vi "Format Aquisition Sequence Array.vi"(8 "Capture/Live":string, 11 "Sequence Cluster Array":T1[](array[typedef]) {"Image Acquisition Parameters"."Z Steps Size (um)" min=0.0; "Image Acquisition Parameters"."Number of Z Steps" min=1; "Image Acquisition Parameters"."Frames Accumulations" min=1; "Image Acquisition Parameters"."Frames Per Capture" min=1; "Image Acquisition Parameters"."Line Accumulations" min=1; "Image Acquisition Parameters"."Image Format" items=["64 x 64"=64, "128 x 128"=128, "256 x 256"=256, "512 x 512"=512, "1024 x 1024"=1024, "2048 x 2048"=2048]; "Laser Parameters"."405 Power (0-5V)" min=0.0 max=5.0}) -> (0 "Channel pixel size array":cluster{i32, i32}[](array[cluster]), 1 "Number of Channels":i32, 2 "Image Acquisition Parameter Array":T2[](array[typedef]) {"Z Steps Size (um)" min=0.0; "Number of Z Steps" min=1; "Frames Accumulations" min=1; "Frames Per Capture" min=1; "Line Accumulations" min=1; "Image Format" items=["64 x 64"=64, "128 x 128"=128, "256 x 256"=256, "512 x 512"=512, "1024 x 1024"=1024, "2048 x 2048"=2048]}, 3 "Detector Parameters Array":T4[](array[typedef]), 4 "Channel Acquisition Parameters Array":T2[](array[typedef]) {"Z Steps Size (um)" min=0.0; "Number of Z Steps" min=1; "Frames Accumulations" min=1; "Frames Per Capture" min=1; "Line Accumulations" min=1; "Image Format" items=["64 x 64"=64, "128 x 128"=128, "256 x 256"=256, "512 x 512"=512, "1024 x 1024"=1024, "2048 x 2048"=2048]})   [LabVIEW 2016]
uses:
  Detectors.ctl
  Type Defs/Image Acquisition Parameters.ctl
  Sequence Cluster_Ctrl.ctl
  Laser Controls.ctl
panel:
  # "Copyright (C) 2020 Edward S Allgeyer\n\nRedistribution and use in source and binary forms, with or without\nmodification, are permitted provided that the following conditions\nare met:\n\n1. Redistributions of source code must retain the above copyright\n   notice, this list of conditions and the following disclaimer.\n\n2. Redistributions in binary form must reproduce the above copyright\n   notice, this list of conditions and the following disclaimer in\n   the documentation and/or other materials provided with the\n   distribution.\n\n3. Neither the name of the copyright holder nor the names of its\n   contributors may be used to endorse or promote products derived\n   from this software without specific prior written permission.\n\nTHIS SOFTWARE IS PROVIDED BY THE COPYRIGHT HOLDERS AND CONTRIBUTORS\n\"AS IS\" AND ANY EXPRESS OR IMPLIED WARRANTIES, INCLUDING, BUT NOT\nLIMITED TO, THE IMPLIED WARRANTIES OF MERCHANTABILITY AND FITNESS\nFOR A PARTICULAR PURPOSE ARE DISCLAIMED. IN NO EVENT SHALL THE\nCOPYRIGHT HOLDER OR CONTRIBUTORS BE LIABLE FOR ANY DIRECT, INDIRECT,\nINCIDENTAL, SPECIAL, EXEMPLARY, OR CONSEQUENTIAL DAMAGES (INCLUDING,\nBUT NOT LIMITED TO, PROCUREMENT OF SUBSTITUTE GOODS OR SERVICES;\nLOSS OF USE, DATA, OR PROFITS; OR BUSINESS INTERRUPTION) HOWEVER\nCAUSED AND ON ANY THEORY OF LIABILITY, WHETHER IN CONTRACT, STRICT\nLIABILITY, OR TORT (INCLUDING NEGLIGENCE OR OTHERWISE) ARISING IN\nANY WAY OUT OF THE USE OF THIS SOFTWARE, EVEN IF ADVISED OF THE\nPOSSIBILITY OF SUCH DAMAGE."
  # "XY"
  # "Z"
  # "Length"
  # "Height"
  # "XY"
  # "Z"
  # "Length"
  # "Height"
  # "XY"
  # "Z"
  # "Length"
  # "Height"
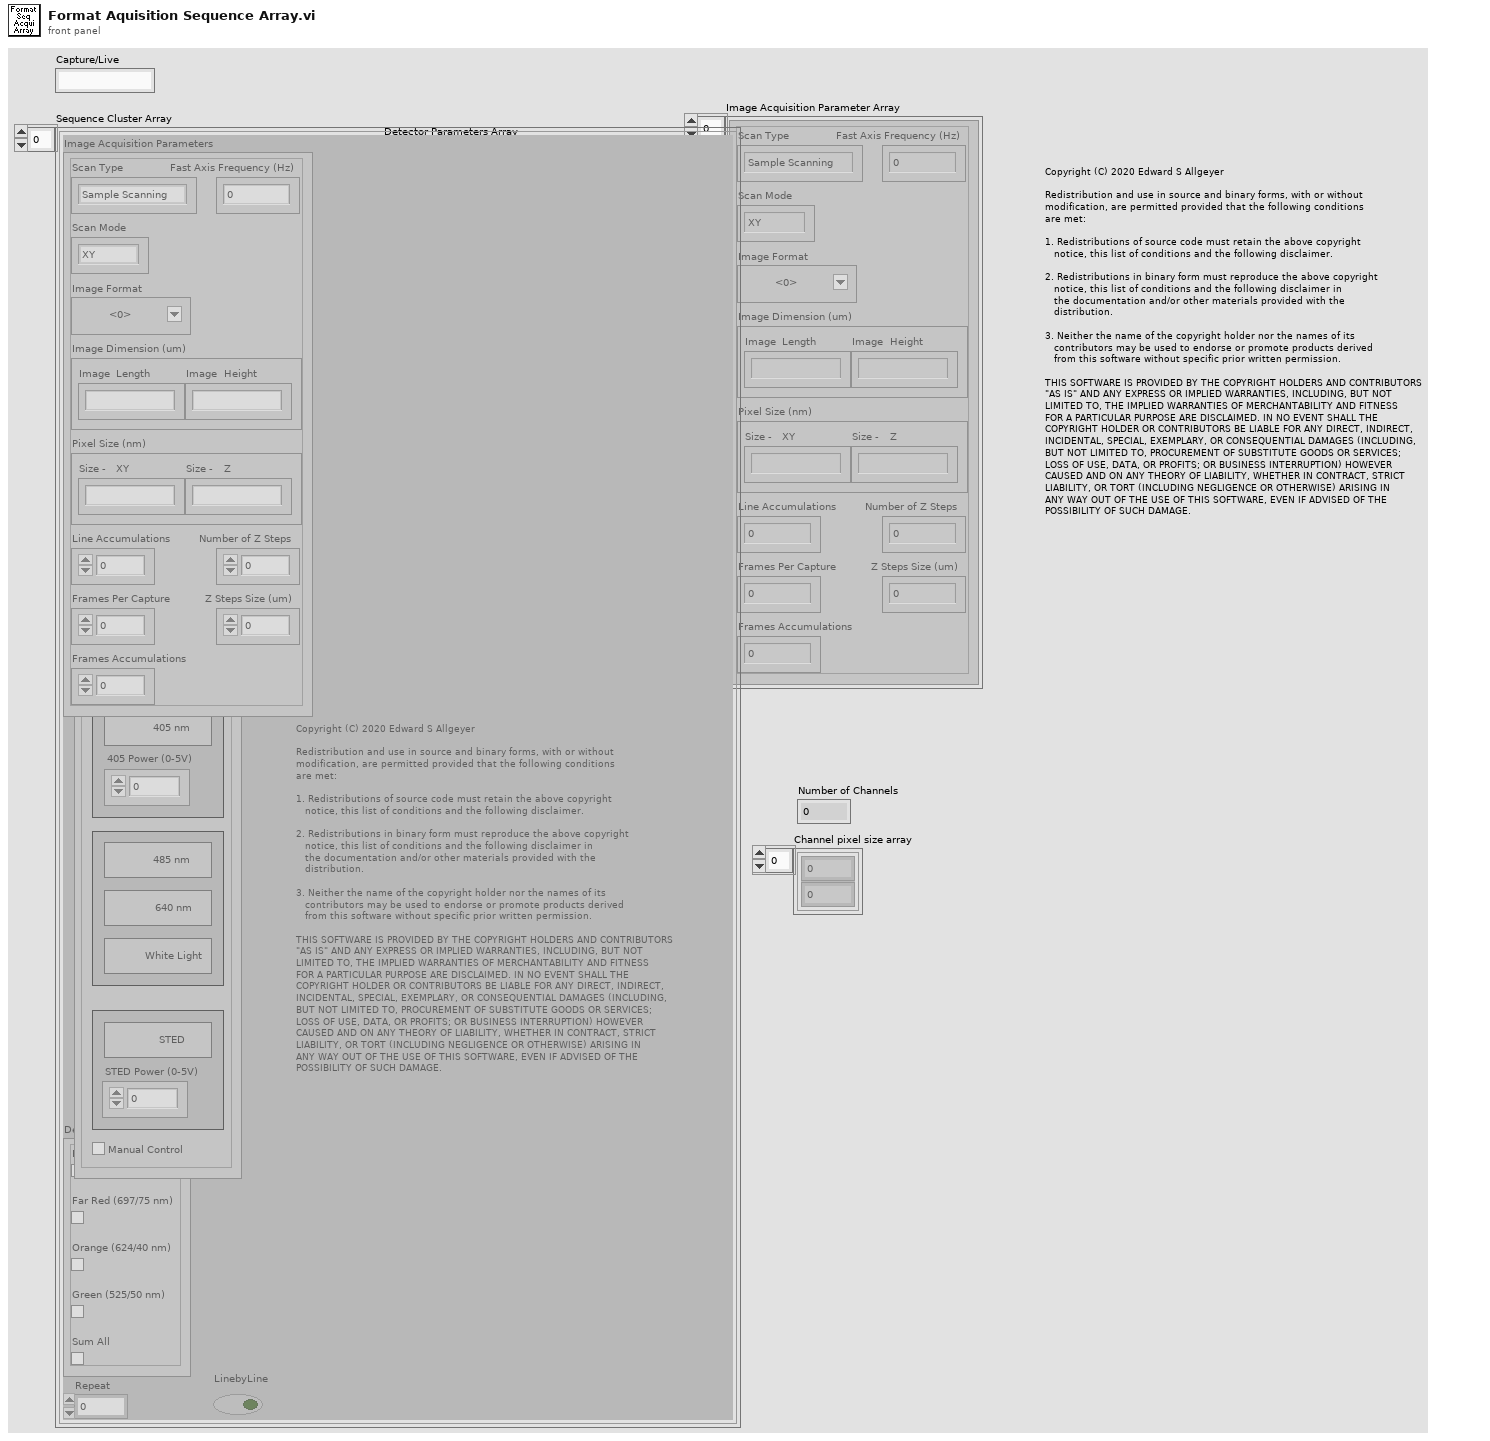
[diagram p1: front panel]
types:
  T1 = typedef "Sequence Cluster_Ctrl.ctl" = cluster{"Image Acquisition Parameters":T2, "Laser Parameters":T3, "Detectors Parameters":T4, "Repeat":dbl, "LinebyLine":bool}
  T2 = typedef "Image Acquisition Parameters.ctl" = cluster{"Scan Type":enum16{"Sample Scanning", "Beam Scanning"}, "Scan Mode":enum16{"XY", "XZ", "YZ", "XYZ"}, "Fast Axis Frequency (Hz)":dbl, "Image Format":u16, "Line Accumulations":u16, "Frames Per Capture":u16, "Frames Accumulations":u16, "Image Dimension (um)":dbl[], "Number of Z Steps":u8, "Z Steps Size (um)":dbl, "Pixel Size (nm)":dbl[]}
  T3 = typedef "Laser Controls.ctl" = cluster{"STED Power (0-5V)":dbl, "STED":bool, "640 nm":bool, "485 nm":bool, "Manual Control":bool, "White Light":bool, "405 nm":bool, "405 Power (0-5V)":dbl}
  T4 = typedef "Detectors.ctl" = cluster{"PMT":bool, "Far Red (697/75 nm)":bool, "Orange (624/40 nm)":bool, "Green (525/50 nm)":bool, "Sum All":bool}
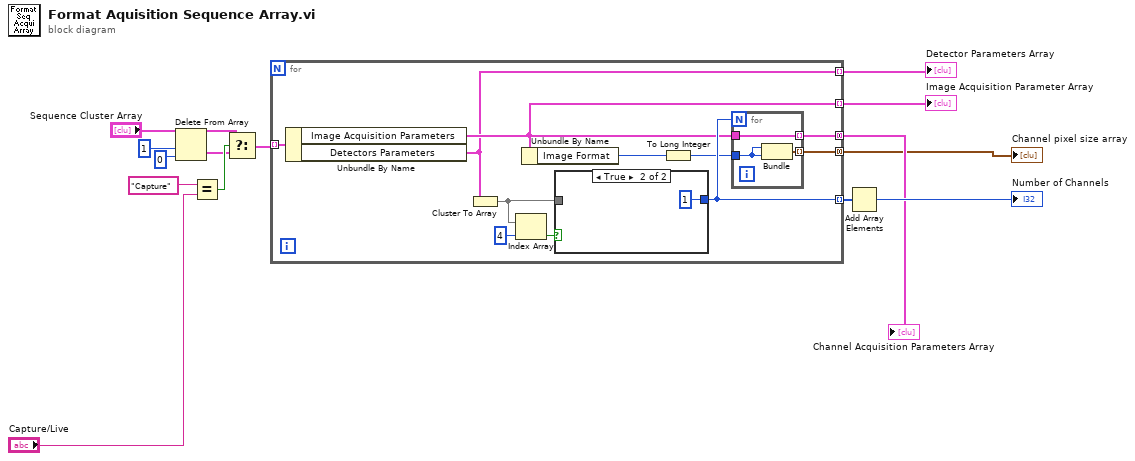
[diagram p0: block diagram]
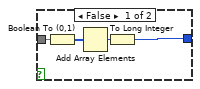
[diagram p2: hidden frame]
diagram:
  n1 = Delete From Array(array="Sequence Cluster Array", length=1, index=0) -> (deleted portion=w9:T1[], array with subset deleted=w8:T1[])
  n2 = Equal?(x="Capture" ("Action"), y="Capture/Live") -> (x = y?=w11:bool)
  n3 = Select(t=w8, s=w11, f=w9) -> (s? t:f=w10:T1[])
  n4 = for {
    tunnel: w10 -> [w26] mode=indexing
    tunnel: [w22] -> w5 mode=concatenating
    tunnel: [w23] -> w4 mode=indexing
    tunnel: [w21] -> w14 mode=indexing
    tunnel: [w20] -> w12 mode=concatenating
    tunnel: [w16] -> w15 mode=indexing
    n5 = Unbundle By Name(w26) -> ("Image Acquisition Parameters"=w21:T2, "Detectors Parameters"=w16:T4)
    n6 = Cluster To Array(cluster=w16) -> (array=w24:bool[])
    n7 = Index Array(array=w24, index=4) -> (element=w17:bool)
    n8 = Unbundle By Name(w21) -> ("Image Format"=w19:u16)
    n9 = case shown="True" w17 {
      tunnel: w24 -> [w30 _]
      tunnel: [w29 1] -> w23
      frame False {
        n10 = Boolean To (0,1)(Boolean=w30) -> (0, 1=w27:i16[])
        n11 = Add Array Elements(numeric array=w27) -> (sum=w28:i16)
        n12 = To Long Integer(number=w28) -> (32bit integer=w29:i32)
      }
      frame True {
      }
    }
    n13 = To Long Integer(number=w19) -> (32bit integer=w18:i32)
    n14 = for {
      N: w23 -> [_]
      tunnel: w18 -> [w34]
      tunnel: [w33] -> w22 mode=indexing
      tunnel: w21 -> [w32]
      tunnel: [w32] -> w20 mode=indexing
      n15 = Bundle(w34, w34) -> (w33:cluster{i32, i32})  [unwired: 1 in]
    }
  }
  "Detector Parameters Array" <- w15
  "Image Acquisition Parameter Array" <- w14
  "Channel Acquisition Parameters Array" <- w12
  "Channel pixel size array" <- w5
  n16 = Add Array Elements(numeric array=w4) -> (sum=→"Number of Channels":i32)
